vi "Main.vi"() -> ()   [LabVIEW 2013]
uses:
  <vilib>/myRIO/Instrument Drivers/Onboard IO/I2C/typedefs/I2C User Configuration.ctl
  <vilib>/myRIO/Instrument Drivers/Onboard IO/I2C/typedefs/I2C Transfer Rate.ctl
  <vilib>/Platform/TimedLoop/XDataNode/timing_clust.ctl
  <vilib>/Platform/TimedLoop/XDataNode/nitl_modes.ctl
  <vilib>/Platform/TimedLoop/XDataNode/wakeup.ctl
  <vilib>/myRIO/Common/Instrument Driver Framework/myRIO v1.0/DIO/vis/myRIO v1.1 Open DIO.vi
  <vilib>/myRIO/Common/Instrument Driver Framework/myRIO v1.0/I2C/vis/myRIO v1.1 Open I2C.vi
  <vilib>/myRIO/Common/Instrument Driver Framework/myRIO v1.0/UART/vis/myRIO v1.0 Close UART.vi
  <vilib>/myRIO/Common/Instrument Driver Framework/Utilities/vis/Validate Channels.vi
  <vilib>/myRIO/Common/Instrument Driver Framework/myRIO v1.0/DIO/vis/myRIO v1.0 Reserve DIO.vi
  <vilib>/myRIO/Common/Instrument Driver Framework/myRIO v1.0/I2C/vis/myRIO v1.0 Reserve I2C.vi
  <vilib>/myRIO/Common/Instrument Driver Framework/myRIO v1.0/Resource Manager/vis/myRIO v1.0 Reserve Channel List.vi
  <vilib>/myRIO/Common/Instrument Driver Framework/myRIO v1.0/DIO/vis/myRIO v1.0 Build MUX Configuration DIO.vi
  <vilib>/myRIO/Common/Instrument Driver Framework/myRIO v1.0/I2C/vis/myRIO v1.0 Build MUX Configuration I2C.vi
  <vilib>/myRIO/Common/Instrument Driver Framework/myRIO v1.0/Resource Manager/vis/myRIO v1.0 Reserve Channel.vi
  <vilib>/myRIO/Common/Instrument Driver Framework/myRIO v1.0/Resource Manager/vis/myRIO v1.0 Unreserve Channel.vi
  <vilib>/myRIO/Common/Instrument Driver Framework/myRIO v1.0/Resource Manager/vis/myRIO v1.0 Create Configuration List.vi
  <vilib>/myRIO/Common/Instrument Driver Framework/myRIO v1.0/Resource Manager/vis/myRIO v1.0 Build Mutex Name.vi
  <vilib>/myRIO/Common/Instrument Driver Framework/myRIO v1.0/myRIO v1.1 Open.vi
  <vilib>/Utility/VariantDataType/GetNumericInfo.vi
  <vilib>/Utility/error.llb/Error Cluster From Error Code.vi
  <vilib>/myRIO/Common/Instrument Driver Framework/Utilities/vis/IO Manager.vi
  <vilib>/myRIO/Common/Instrument Driver Framework/Utilities/vis/Configuration Manager.vi
  <vilib>/myRIO/Common/Instrument Driver Framework/myRIO v1.0/Resource Manager/vis/myRIO v1.0 Configure IO.vi
  <vilib>/myRIO/Common/Instrument Driver Framework/myRIO v1.0/myRIO v1.0 Close.vi
  <vilib>/myRIO/Common/Instrument Driver Framework/myRIO v1.0/I2C/vis/myRIO v1.0 Configure I2C.vi
  <vilib>/myRIO/Common/Instrument Driver Framework/myRIO v1.0/I2C/vis/myRIO v1.0 Write I2C.vi
  <vilib>/myRIO/Common/Instrument Driver Framework/myRIO v1.0/DIO/vis/myRIO v1.0 Read DIO.vi
  <vilib>/myRIO/Common/Instrument Driver Framework/myRIO v1.0/DIO/vis/myRIO v1.0 Write DIO.vi
  <vilib>/myRIO/Common/Instrument Driver Framework/myRIO v1.0/I2C/vis/myRIO v1.0 Read I2C.vi
  <vilib>/myRIO/Common/Instrument Driver Framework/Utilities/vis/FPGA Ref Manager.vi
  <vilib>/myRIO/Common/Instrument Driver Framework/myRIO v1.0/myRIO v1.0 Reset FPGA.vi
  <vilib>/platform/TimedLoop/XDataNode/XDataNode.xnode
  <vilib>/myRIO/Instrument Drivers/Utilities/Utilities.lvlib
  <vilib>/myRIO/Instrument Drivers/Onboard IO/I2C/I2C.lvlib
  <vilib>/myRIO/Instrument Drivers/Onboard IO/DIO/DIO.lvlib
  <vilib>/Platform/TimedLoop/XDataNode/XDNodeRunTimeDep.lvlib
panel:
  out "Angular rate [LSB/sec]":cluster{i16, i16, i16}(graph)
  out "DATA":u8[](array[numeric]) format="%02x"
  out "Z rate":i16
  out "Y rate":i16
  out "X rate":i16
  in  "[ESC]":bool
  # "Gyroscope demo"
  # "OUT_X_L"
  # "OUT_X_H"
  # "OUT_Y_L"
  # "OUT_Y_H"
  # "OUT_Z_L"
  # "OUT_Z_H"
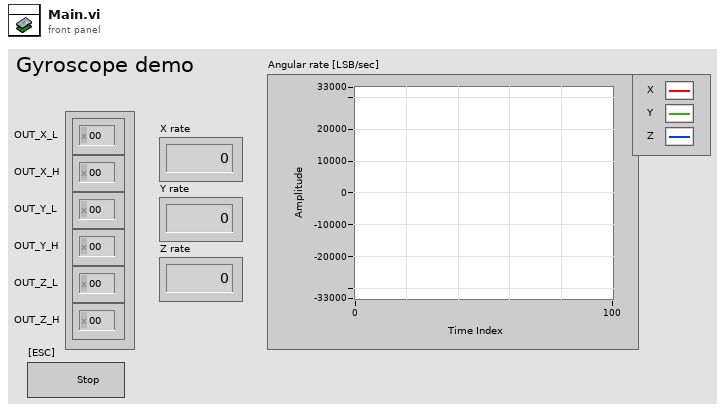
[diagram p1: front panel]
types:
  T1 = typedef "I2C.lvlib/I2C User Configuration.ctl" = cluster{"I2C Transfer Rate":T2}
  T2 = typedef "I2C.lvlib/I2C Transfer Rate.ctl" = enum16{"Standard Mode (100 kbps)", "Fast Mode (400 kbps)"}
  T3 = typedef "I2C.lvlib/I2C Reference.ctl" = cluster{"myRIO Reference":T4, "I2C Channels Enum":T8, "I2C Configuration":T9}
  T4 = typedef "myRIO Generic Hardware Reference.ctl" = cluster{"myRIO Model":T5, "myRIO Hardware Reference":T6}
  T5 = typedef "Hardware Version Enum.ctl" = enum16{"Unknown", "myRIO-1900", "myRIO-1950"}
  T6 = typedef "myRIO v1.0 Reference.ctl" = cluster{"Generic FPGA Reference":T7, "Allow multiple opens":bool}
  T7 = typedef "Generic FPGA Reference.ctl" = refnum<k20>
  T8 = typedef "I2C Channels Enum.ctl" = enum16{"Not Connected", "A/I2C", "B/I2C"}
  T9 = typedef "I2C.lvlib/I2C Configuration.ctl" = cluster{"I2C Transfer Rate":T2}
  T10 = typedef "DIO.lvlib/DIO Reference.ctl" = cluster{"myRIO Reference":T4, "DIO Channels List":T11}
  T11 = typedef "DIO Channels List.ctl" = T12[]
  T12 = typedef "DIO Channels Enum.ctl" = enum16{"Not Connected", "C/DIO0", "C/DIO1", "C/DIO2", "C/DIO3", "C/DIO4", "C/DIO5", "C/DIO6", "C/DIO7", "A/DIO0", "A/DIO1", "A/DIO2", "A/DIO3", "A/DIO4", "A/DIO5", "A/DIO6", "A/DIO7", "A/DIO8", "A/DIO9", "A/DIO10", "A/DIO11", "A/DIO12", "A/DIO13", "A/DIO14", "A/DIO15", "B/DIO0", "B/DIO1", "B/DIO2", "B/DIO3", "B/DIO4", "B/DIO5", "B/DIO6", "B/DIO7", "B/DIO8", "B/DIO9", "B/DIO10", "B/DIO11", "B/DIO12", "B/DIO13", "B/DIO14", "B/DIO15", "LED0", "LED1", "LED2", "LED3", "Button0"}
  T13 = typedef "XDNodeRunTimeDep.lvlib/timing_clust.ctl" = cluster{"Expected End [f-1]":u64, "Actual End [f-1]":u64, "Finished Late? [f-1]":bool, "Expected End [i-1]":u64, "Actual End [i-1]":u64, "Finished Late? [i-1]":bool, "Expected Start [i]":u64, "Actual Start [i]":u64, "Expected Start [f]":u64, "Actual Start [f]":u64, "Source Name":string, "Structure Name":string, "Period":i64, "Deadline":i64, "Offset":i64, "Start":i64, "Priority":i32, "Timeout":i32, "Mode":T14, "Wakeup Reason":T15, "Error":errorcluster, "Source Type":string, "Secondary Source Type":string, "Global End Time":u64, "Global Start Time":u64, "Frame Duration":u64, "Iteration Duration":u64, "Assigned CPU":i32, "I/O Scan Engine Mode":u32}
  T14 = typedef "XDNodeRunTimeDep.lvlib/nitl_modes.ctl" = enum32{"No Change", "Process missed periods, maintain original phase", "Discard missed periods, maintain original phase", "Process missed periods, ignore original phase", "Discard missed periods, ignore original phase"}
  T15 = typedef "XDNodeRunTimeDep.lvlib/wakeup.ctl" = enum32{"Normal", "Aborted", "Asynchronous wakeup", "Timing source error", "Timed loop error", "Timeout"}
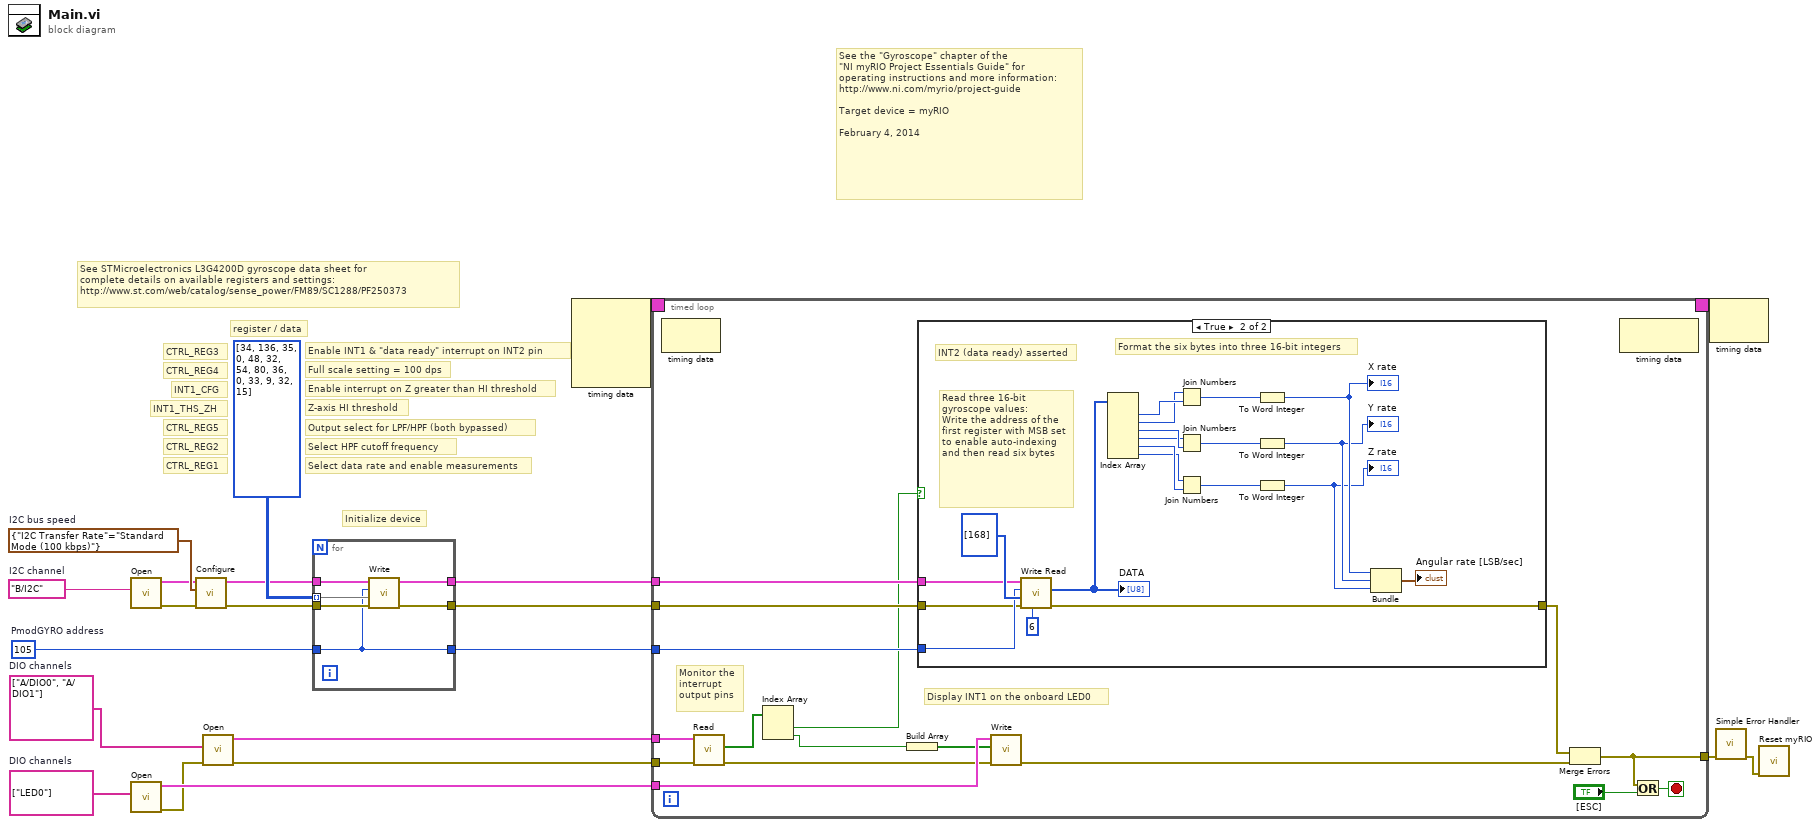
[diagram p0: block diagram]
diagram:
  w3 = tag[] ["LED0"]  # DIO channels
  w6 = tag[] ["A/DIO0", "A/DIO1"]  # DIO channels
  w18 = T1 {"I2C Transfer Rate"=enum."Standard Mode (100 kbps)"}  # I2C bus speed
  w19 = tag "B/I2C"  # I2C channel
  w9 = u8 105  # PmodGYRO address
  # "See the \"Gyroscope\" chapter of the\n\"NI myRIO Project Essentials Guide\" for\noperating instructions and more information: \nhttp://www.ni.com/myrio/project-guide\n\nTarget device = myRIO\n\nFebruary 4, 2014"
  # "Enable INT1 & \"data ready\" interrupt on INT2 pin"
  # "CTRL_REG3"
  # "Select HPF cutoff frequency"
  # "CTRL_REG2"
  # "Output select for LPF/HPF (both bypassed)"
  # "CTRL_REG5"
  # "Initialize device"
  # "Select data rate and enable measurements"
  # "Z-axis HI threshold"
  # "Enable interrupt on Z greater than HI threshold"
  # "See STMicroelectronics L3G4200D gyroscope data sheet for\ncomplete details on available registers and settings:\nhttp://www.st.com/web/catalog/sense_power/FM89/SC1288/PF250373"
  # "CTRL_REG1"
  # "INT1_THS_ZH"
  # "INT1_CFG"
  # "Full scale setting = 100 dps"
  # "CTRL_REG4"
  # "register / data"
  n1 = call <vilib>:"Open.vi"("Channel Name"=w19) -> ("error out"=w16:errorcluster, "I2C Ref Out"=w17:T3)  [unwired: 9 in]
  n2 = call <vilib>:"Open.vi"("Channel Names"=w3) -> ("error out"=w1:errorcluster, "DIO Ref Out"=w2:T10)  [unwired: 9 in]
  n3 = call <vilib>:"Configure.vi"("error in (no error)"=w16, "I2C User Configuration"=w18, "I2C Ref In"=w17) -> ("error out"=w10:errorcluster, "I2C Ref Out"=w11:T3)  [unwired: 7 in]
  n4 = call <vilib>:"Open.vi"("error in (no error)"=w1, "Channel Names"=w6) -> ("error out"=w8:errorcluster, "DIO Ref Out"=w7:T10)  [unwired: 8 in]
  n5 = for {
    tunnel: [w27] -> w15
    tunnel: [w26] -> w14
    tunnel: [w22] -> w13
    tunnel: u8[][] [[34, 136], [35, 0], [48, 32], [54, 80], [36, 0], [33, 9], [32, 15]] ("Bytes to Write") -> [w25] mode=indexing
    tunnel: w11 -> [w24]
    tunnel: w10 -> [w23]
    tunnel: w9 -> [w22]
    n6 = call <vilib>:"Write.vi"("error in (no error)"=w23, "Bytes to Write"=w25, "Slave Address (7-bit)"=w22, "I2C Ref In"=w24) -> ("error out"=w27:errorcluster, "I2C Ref Out"=w26:T3)  [unwired: 6 in]
  }
  n7 = node-c288() -> (w5:T13)  [unwired: 4 in]
  n8 = timed-loop {
    tunnel: [w28] -> w20
    tunnel: w13 -> [w39]
    tunnel: w15 -> [w41]
    tunnel: w14 -> [w40]
    tunnel: w8 -> [w38]
    tunnel: w7 -> [w37]
    timing: w5 -> [_]
    timing-out: [_] -> w4
    tunnel: w2 -> [w33]
    stop <- w43 stop-if-true
    # "Display INT1 on the onboard LED0"
    # "Monitor the\ninterrupt\noutput pins"
    n9 = node-c288() -> ()  [unwired: 1 in, 1 out]
    n10 = call <vilib>:"Read.vi"("error in (no error)"=w38, "DIO Ref In"=w37) -> ("error out"=w32:errorcluster, "Values"=w34:bool[])  [unwired: 7 in, 1 out]
    n11 = Index Array "Index Array"(array=w34) -> (element #1=w35:bool, element #2=w30:bool)  [unwired: 2 in]
    n12 = Build Array "Build Array"(w30) -> (w31:bool[])
    n13 = case shown="True" w35 {
      tunnel: w41 -> [w46 w47]
      tunnel: w40 -> [_ w48]
      tunnel: w39 -> [_ w54]
      tunnel: [w46 w53] -> w36
      frame False {
        # "INT2 (data ready) deasserted"
      }
      frame True {
        # "INT2 (data ready) asserted"
        # "Read three 16-bit gyroscope values:\nWrite the address of the first register with MSB set to enable auto-indexing and then read six bytes"
        # "Format the six bytes into three 16-bit integers"
        n14 = call <vilib>:"Write Read.vi"("Byte Count"=u32 6, "error in (no error)"=w47, "Bytes to Write"=u8[] [168], "Slave Address (7-bit)"=w54, "I2C Ref In"=w48) -> ("error out"=w53:errorcluster, "Bytes Read"=w52:u8[])  [unwired: 3 in, 1 out]
        "DATA" <- w52
        n15 = Index Array "Index Array"(array=w52) -> (element #1=w62:u8, element #2=w61:u8, element #3=w60:u8, element #4=w59:u8, element #5=w58:u8, element #6=w57:u8)  [unwired: 6 in]
        n16 = Join Numbers(hi=w61, lo=w62) -> ((hi.lo)=w66:u16)
        n17 = Join Numbers(hi=w59, lo=w60) -> ((hi.lo)=w65:u16)
        n18 = Join Numbers(hi=w57, lo=w58) -> ((hi.lo)=w64:u16)
        n19 = To Word Integer(number=w66) -> (16bit integer=w51:i16)
        "X rate" <- w51
        n20 = To Word Integer(number=w65) -> (16bit integer=w50:i16)
        "Y rate" <- w50
        n21 = To Word Integer(number=w64) -> (16bit integer=w49:i16)
        "Z rate" <- w49
        n22 = Bundle "Bundle"(w51, w50, w49) -> (→"Angular rate [LSB/sec]":cluster{i16, i16, i16})  [unwired: 1 in]
      }
    }
    n23 = call <vilib>:"Write.vi"("error in (no error)"=w32, "Values"=w31, "DIO Ref In"=w33) -> ("error out"=w29:errorcluster)  [unwired: 6 in, 1 out]
    n24 = Merge Errors "Merge Errors"(w36, w29) -> (w28:errorcluster)
    n25 = node-c288() -> ()  [unwired: 1 in, 1 out]
    n26 = Or(x=w28, y="[ESC]") -> (x .or. y?=w43:bool)
  }
  n27 = node-c288(w4) -> ()  [unwired: 1 out]
  n28 = call <vilib>:"Simple Error Handler.vi"("error in (no error)"=w20) -> ("error out"=w21:errorcluster)  [unwired: 4 in, 4 out]
  n29 = call <vilib>:"Reset myRIO.vi"("error in (no error)"=w21) -> ()  [unwired: 10 in, 1 out]
